vi "G.vi"(8 "error in (no error)":errorcluster caption="エラー入力（エラーなし）", 9 "distance":u32, 10 "direction (+/-)":string, 11 "VISAリソース名":refnum<visa-resource-name>) -> (0 "error out":errorcluster caption="エラー出力", 3 "VISAリソース名（出力）":refnum<visa-resource-name>)   [LabVIEW 2017]
panel:
  in  "文字入力待機 (100 ms)":u16=100
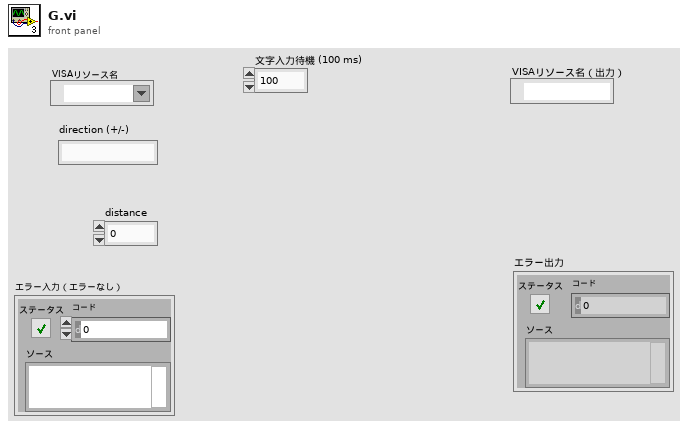
[diagram p1: front panel]
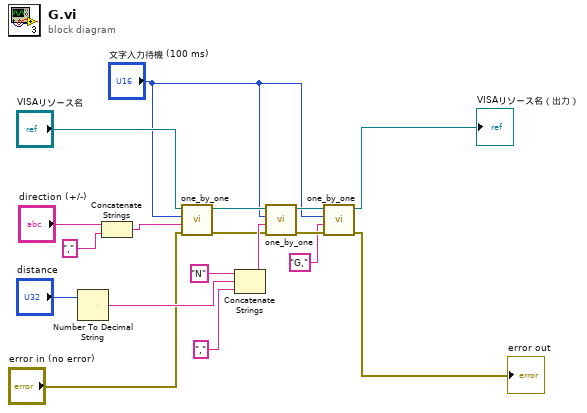
[diagram p0: block diagram]
diagram:
  n1 = Number To Decimal String(number="distance") -> (decimal integer string=w8:string)  [unwired: 1 in]
  n2 = Concatenate Strings("direction (+/-)", ",") -> (w2:string)
  n3 = call "one_by_one.vi"("error in (no error)"="error in (no error)", "入力文字"=w2, "待機 (200ms)"="文字入力待機 (100 ms)", "VISAリソース名"="VISAリソース名") -> ("error out"=w15:errorcluster, "VISAリソース名出力"=w17:refnum<visa-resource-name>)  [unwired: 6 in]
  n4 = Concatenate Strings("N", w8, ",") -> (w16:string)
  n5 = call "one_by_one.vi"("error in (no error)"=w15, "入力文字"=w16, "待機 (200ms)"="文字入力待機 (100 ms)", "VISAリソース名"=w17) -> ("error out"=w14:errorcluster, "VISAリソース名出力"=w13:refnum<visa-resource-name>)  [unwired: 6 in]
  n6 = call "one_by_one.vi"("error in (no error)"=w14, "入力文字"="G,", "待機 (200ms)"="文字入力待機 (100 ms)", "VISAリソース名"=w13) -> ("error out"=→"error out":errorcluster, "VISAリソース名出力"=→"VISAリソース名（出力）":refnum<visa-resource-name>)  [unwired: 6 in]
